vi "Datasocket(Sin)服务器.vi"() -> ()   [LabVIEW 2017]
uses:
  <vilib>/Analysis/NI_AALBase.lvlib
panel:
  in  "停止":bool
  out "波形图":dbl[](graph)
  in  "cycles":dbl=1.0 caption="周期" format="%0.2f"
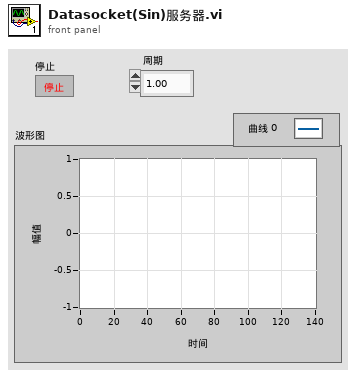
[diagram p1: front panel]
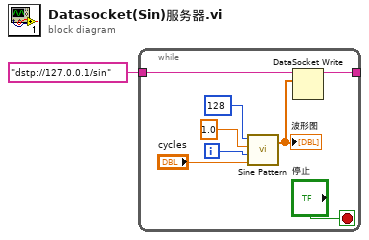
[diagram p0: block diagram]
diagram:
  n1 = while {
    tunnel: "dstp://127.0.0.1/sin" ("连接输入") -> [w9]
    tunnel: [w5] -> _
    i -> [w8]
    stop <- "停止" stop-if-true
    n2 = call <vilib>:"Sine Pattern.vi"("cycles"="cycles", "phase(degrees)"=w8, "amplitude"=1.0, "samples"=128) -> ("Sinusoidal Pattern"=w3:dbl[])  [unwired: 1 out]
    "波形图" <- w3
    n3 = DataSocket Write(10:w3, 11:w9) -> (3:w5:string)  [unwired: 2 in, 2 out]
  }
